vi "3DMotion.vi"(6 "phi":dbl, 9 "psi":dbl, 10 "th":dbl, 11 "SceneObject in":refnum<vi>) -> ()   [LabVIEW 2017]
uses:
  <vilib>/picture/3D Picture Control/NI_3D Picture Control.lvlib
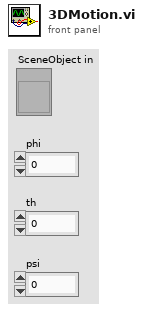
[diagram p1: front panel]
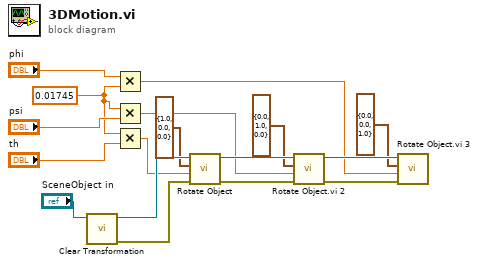
[diagram p0: block diagram]
diagram:
  w2 = 0.01745 ("x")
  n1 = call <vilib>:"Clear Transformation.vi"("Object Refnum In"="SceneObject in") -> ("error out"=w13:errorcluster, "Object Refnum Out"=w14:refnum<vi>)  [unwired: 9 in]
  n2 = Multiply(x="phi", y=w2) -> (x*y=w5:dbl)
  n3 = Multiply(x=w2, y="psi") -> (x*y=w4:dbl)
  n4 = Multiply(x=w2, y="th") -> (x*y=w3:dbl)
  n5 = call <vilib>:"Rotate Object.vi"("error in (no error)"=w13, "Angle"=w3, "Axis"=cluster{"X":sgl, "Y":sgl, "Z":sgl} {"X"=1.0, "Y"=0.0, "Z"=0.0}, "Scene.Object In"=w14) -> ("error out"=w9:errorcluster, "Scene.Object Out"=w12:refnum<vi>)  [unwired: 6 in]
  n6 = call "Rotate Object.vi 2"("error in (no error)"=w9, "Angle"=w4, "Axis"=cluster{"X":sgl, "Y":sgl, "Z":sgl} {"X"=0.0, "Y"=1.0, "Z"=0.0}, "Scene.Object In"=w12) -> ("error out"=w10:errorcluster, "Scene.Object Out"=w11:refnum<vi>)  [unwired: 6 in]
  n7 = call "Rotate Object.vi 3"("error in (no error)"=w10, "Angle"=w5, "Axis"=cluster{"X":sgl, "Y":sgl, "Z":sgl} {"X"=0.0, "Y"=0.0, "Z"=1.0}, "Scene.Object In"=w11) -> ()  [unwired: 6 in, 2 out]
